vi "RampUpMkI.vi"() -> ()   [LabVIEW 2010]
uses:
  <vilib>/FTC/FTC ControllerState.ctl
  <vilib>/FTC/FTC POVState.ctl
  <vilib>/NXT/Dual Mode Library/prims/inRangeAndCoerce/inRangeAndCoerce_int.vi
panel:
  in  "Time Span":i32=10
  in  "Left Y":i32=100
  out "Power out":i32
  in  "Controller State 2":T1={"Left X"=0, "Left Y"=0, "Right X"=0, "Right Y"=0, "Button Encoding 9-12"=0, "Button Encoding 1-8"=0, "POV"=-1} {"POV" items=["None"=-1, "POV Up"=0, "POV Up Right"=1, "POV Right"=2, "POV Down Right"=3, "POV Down"=4, "POV Down Left"=5, "POV Left"=6, "POV Up Left"=7]}
  out "Controller State":T1={"Left X"=0, "Left Y"=0, "Right X"=0, "Right Y"=0, "Button Encoding 9-12"=0, "Button Encoding 1-8"=0, "POV"=-1} {"POV" items=["None"=-1, "POV Up"=0, "POV Up Right"=1, "POV Right"=2, "POV Down Right"=3, "POV Down"=4, "POV Down Left"=5, "POV Left"=6, "POV Up Left"=7]}
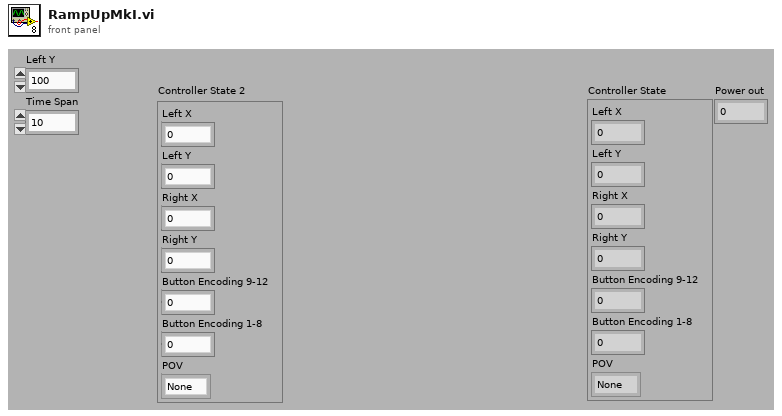
[diagram p1: front panel]
types:
  T1 = typedef "FTC ControllerState.ctl" = cluster{"Left X":i8, "Left Y":i8, "Right X":i8, "Right Y":i8, "Button Encoding 9-12":u8, "Button Encoding 1-8":u8, "POV":T2}
  T2 = typedef "FTC POVState.ctl" = i8
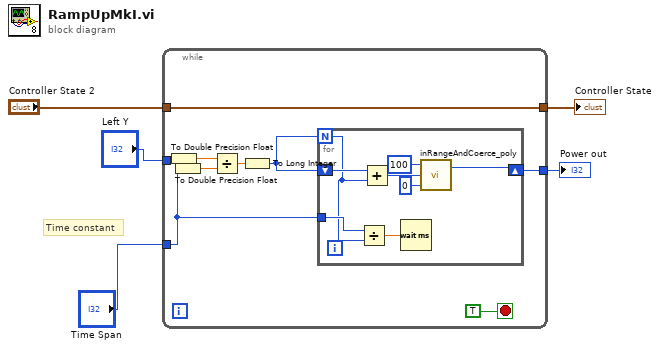
[diagram p0: block diagram]
diagram:
  # "Time constant"
  n1 = while {
    tunnel: "Controller State 2" -> [w13]
    tunnel: [w13] -> w4
    tunnel: "Time Span" -> [w6]
    tunnel: "Left Y" -> [w12]
    tunnel: [w7] -> w1
    stop <- TRUE stop-if-true
    n2 = To Double Precision Float(number=w12) -> (double precision float=w10:dbl)
    n3 = To Double Precision Float(number=w6) -> (double precision float=w9:dbl)
    n4 = Divide(x=w10, y=w9) -> (x/y=w11:dbl)
    n5 = To Long Integer(number=w11) -> (32bit integer=w8:i32)
    n6 = for {
      N: w8 -> [w20]
      shift-right: [w17] -> w7
      shift-left: w8 -> [w22]
      tunnel: w6 -> [w21]
      n7 = Divide(x=w21, y=w20) -> (x/y=w19:dbl)
      n8 = Add(x=w22, y=w20) -> (x+y=w18:i32)
      n9 = Wait (ms)(milliseconds to wait=w19) -> ()  [unwired: 1 out]
      n10 = call-poly <vilib>:"inRangeAndCoerce_poly.vi"("lower limit"=0, "x"=w18, "upper limit"=100) -> ("coerced(x)"=w17:i32)  [unwired: 1 out]
    }
  }
  "Controller State" <- w4
  "Power out" <- w1
